vi "Tracepoint_Init.vi"(8 "error in (no error)":errorcluster, 10 "config":T1, 11 "Qbus":refnum<class "Qbus.lvclass">) -> (0 "error out":errorcluster)   [LabVIEW 2017, in "FileManager.lvlib"]
uses:
  <vilib>/addons/InsightCM/Devices/Shared/Common/FileManager/FileManager.lvlib
  <vilib>/addons/Qbus/Qbus.lvclass
  <vilib>/addons/InsightCM/Devices/Shared/Common/FileManager/controls/config.ctl
  <vilib>/addons/TraceLogger/TraceLogger.lvlib
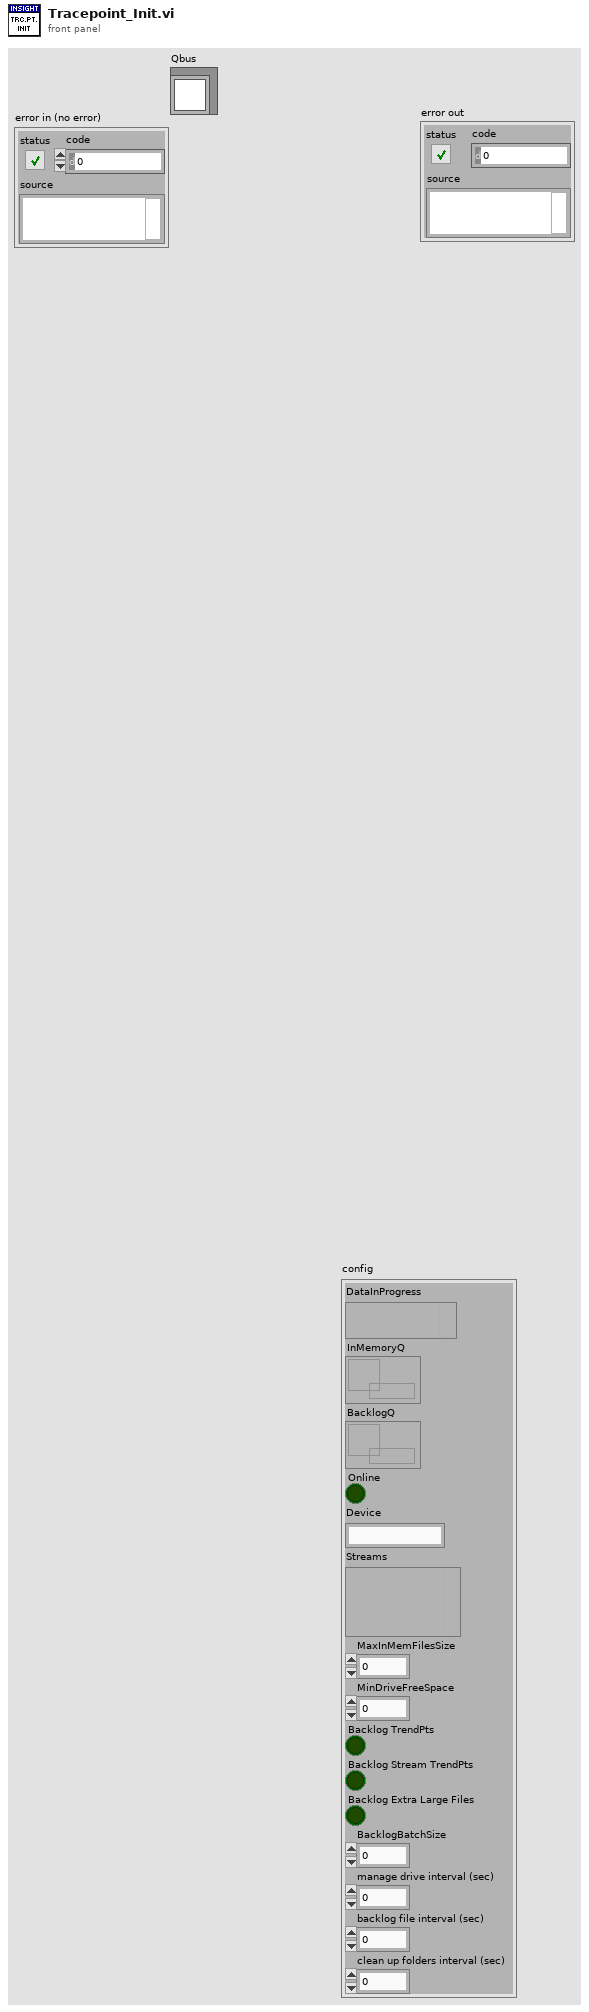
[diagram p1: front panel]
types:
  T1 = typedef "FileManager.lvlib/config.ctl" = cluster{"DataInProgress":variant, "InMemoryQ":refnum<queue>, "BacklogQ":refnum<queue>, "Online":bool, "Device":string, "Streams":variant, "MaxInMemFilesSize":i32, "MinDriveFreeSpace":i32, "Backlog TrendPts":bool, "Backlog Stream TrendPts":bool, "Backlog Extra Large Files":bool, "BacklogBatchSize":i32, "manage drive interval (sec)":dbl, "backlog file interval (sec)":dbl, "clean up folders interval (sec)":dbl}
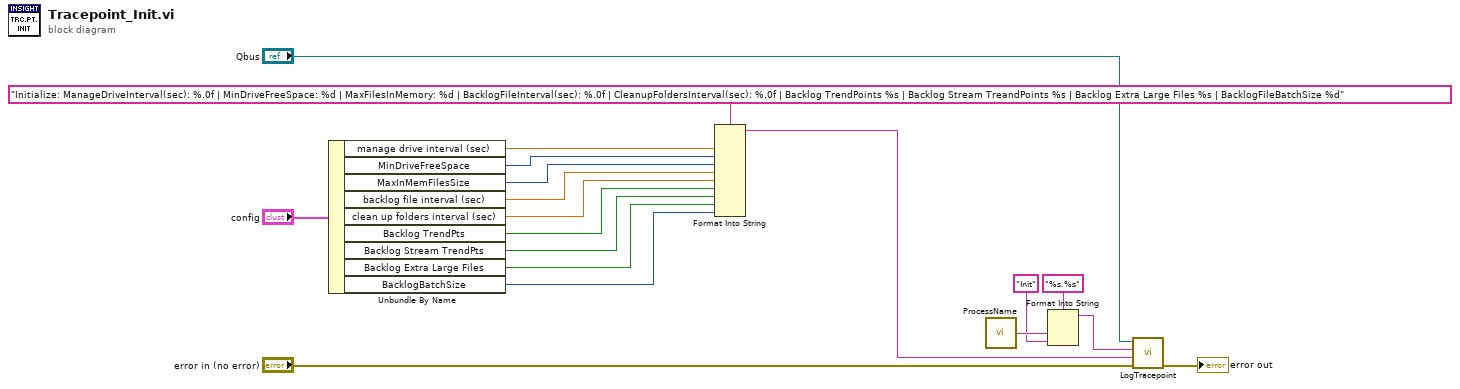
[diagram p0: block diagram]
diagram:
  n1 = Unbundle By Name("config") -> ("manage drive interval (sec)"=w9:dbl, "MinDriveFreeSpace"=w8:i32, "MaxInMemFilesSize"=w7:i32, "backlog file interval (sec)"=w6:dbl, "clean up folders interval (sec)"=w5:dbl, "Backlog TrendPts"=w4:bool, "Backlog Stream TrendPts"=w3:bool, "Backlog Extra Large Files"=w2:bool, "BacklogBatchSize"=w1:i32)
  n2 = Format Into String(format string="Initialize: ManageDriveInterval(sec): %.0f | MinDriveFreeSpace: %d | MaxFilesInMemory: %d | BacklogFileInterval(sec): %.0f | CleanupFoldersInterval(sec): %.0f | Backlog TrendPoints %s | Backlog Stream TreandPoints %s | Backlog Extra Large Files %s | BacklogFileBatchSize %d", w9, w8, w7, w6, w5, w4, w3, w2, w1) -> (resulting string=w11:string)  [unwired: 2 in, 1 out]
  n3 = call <vilib>:"ProcessName.vi"() -> ("process name"=w18:string)  [unwired: 5 in]
  n4 = Format Into String(format string="%s.%s", w18, "Init" ("tracepoint")) -> (resulting string=w15:string)  [unwired: 2 in, 1 out]
  n5 = call <vilib>:"LogTracepoint.vi"("error in (no error)"="error in (no error)", "log string"=w11, "tracepoint"=w15, "qbus in"="Qbus") -> ("error out"=→"error out":errorcluster)  [unwired: 6 in, 1 out]
